vi "MailNum2SQLSubVI.vi"(1 "mail numbers":string) -> (0 "String":string)   [LabVIEW 2011]
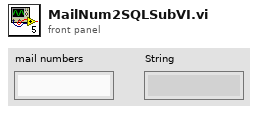
[diagram p1: front panel]
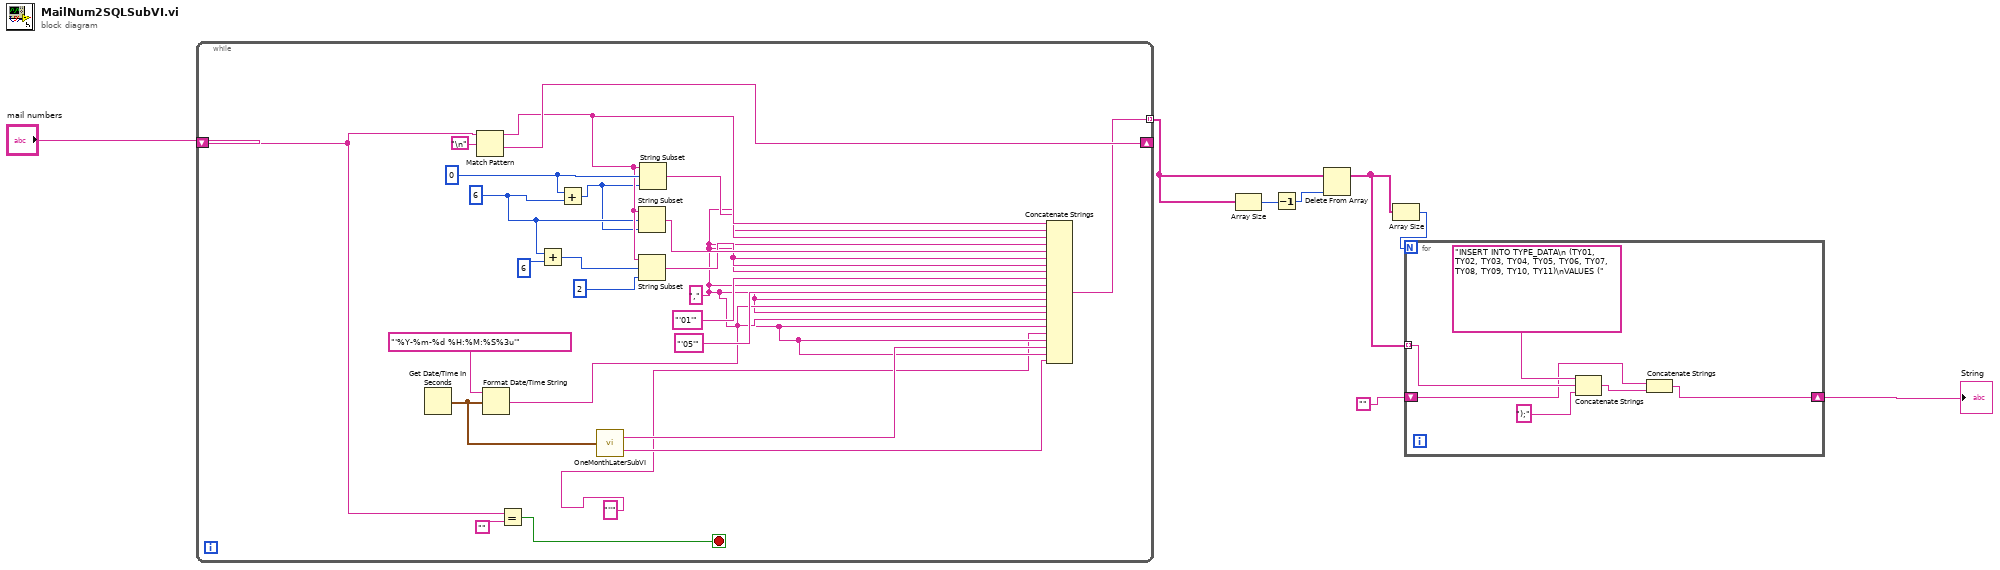
[diagram p0: block diagram]
diagram:
  n1 = while {
    tunnel: [w22] -> w2 mode=indexing
    shift-right: [w30] -> _
    shift-left: "mail numbers" -> [w31]
    stop <- w32 stop-if-true
    w11 = ","
    w21 = 6 ("y")
    w28 = 0 ("offset (0)")
    n2 = Get Date/Time In Seconds() -> (seconds since 1Jan1904=w13:timestamp)
    n3 = Match Pattern(string=w31, regular expression="\n") -> (before substring=w26:string, after substring=w30:string)  [unwired: 1 in, 2 out]
    n4 = Format Date/Time String(time format string (%c)="'%Y-%m-%d %H:%M:%S%3u'", seconds (now)=w13) -> (date/time string=w14:string)  [unwired: 1 in]
    n5 = Equal?(x=w31, y="") -> (x = y?=w32:bool)
    n6 = Add(x=w21, y=6) -> (x+y=w20:i32)
    n7 = Add(x=w28, y=w21) -> (x+y=w18:i32)
    n8 = call "OneMonthLaterSubVI.vi"("timestamp"=w13) -> ("current date"=w12:string, "one month later date"=w10:string)
    n9 = String Subset(string=w26, offset (0)=w21, length (rest)=w18) -> (substring=w24:string)
    n10 = String Subset(string=w26, offset (0)=w20, length (rest)=2 ("y")) -> (substring=w23:string)
    n11 = String Subset(string=w26, offset (0)=w28, length (rest)=w18) -> (substring=w25:string)
    n12 = Concatenate Strings(w26, w11, w25, w11, w24, w11, w23, w11, "'01'", w11, "'05'", w11, w14, w11, w14, w11, "''", w11, w12, w11, w10) -> (w22:string)
  }
  n13 = Array Size(array=w2) -> (size(s)=w3:i32)
  n14 = Decrement(x=w3) -> (x-1=w4:i32)
  n15 = Delete From Array(array=w2, index=w4) -> (array with subset deleted=w6:string[])  [unwired: 1 in, 1 out]
  n16 = Array Size(array=w6) -> (size(s)=w7:i32)
  n17 = for {
    N: w7 -> [_]
    tunnel: w6 -> [w39] mode=indexing
    shift-right: [w34] -> w8
    shift-left: "" -> [w36]
    n18 = Concatenate Strings("INSERT INTO TYPE_DATA\n (TY01, TY02, TY03, TY04, TY05, TY06, TY07, TY08, TY09, TY10, TY11)\nVALUES (" ("string"), w39, ");") -> (w35:string)
    n19 = Concatenate Strings(w36, w35) -> (w34:string)
  }
  "String" <- w8
